vi "List Controls.vi"(8 "error in (no error)":errorcluster, 11 "Rename in":refnum<class "ProjectItem.lvclass">) -> (0 "error out":errorcluster, 3 "Rename out":refnum<class "ProjectItem.lvclass">)   [LabVIEW 2019, in "ProjectItem.lvclass"]
uses:
  ProjectItem.lvclass
  ProjectItem.lvclass/ProjectItem.ctl
  <vilib>/regexp/Match Regular Expression.xnode
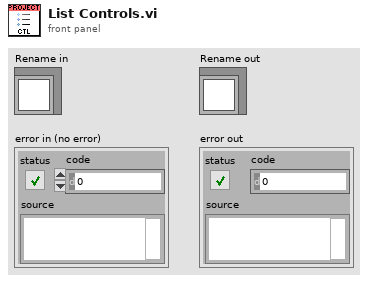
[diagram p1: front panel]
types:
  T1 = cluster{"Class":refnum<vi>, "DynamicVIs":refnum<vi>[], "StaticVIs":refnum<vi>[], "Controls":refnum<vi>[], "Name":string, "Icon":refnum<class "Icon.lvclass">}[]
  T2 = cluster{"Class":refnum<vi>, "DynamicVIs":refnum<vi>[], "StaticVIs":refnum<vi>[], "Controls":refnum<vi>[], "Name":string, "Icon":refnum<class "Icon.lvclass">}
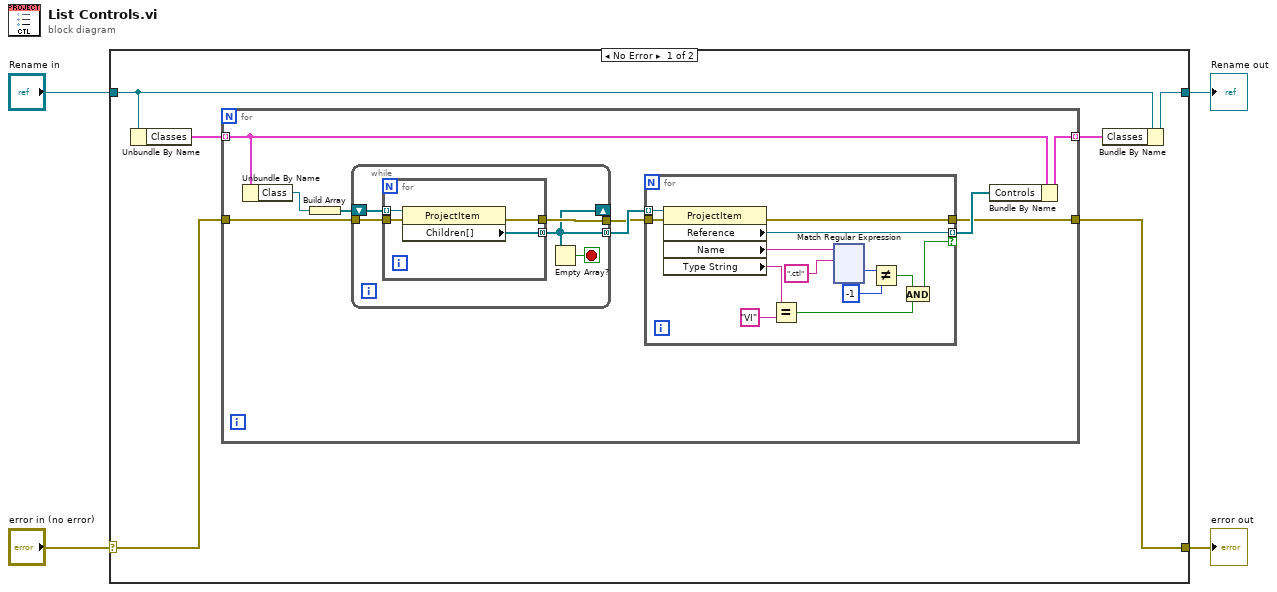
[diagram p0: block diagram]
diagram:
  n1 = case shown="No Error" "error in (no error)" {
    selector: "error in (no error)" -> [w6 w157]
    tunnel: [w9 w156] -> w4
    tunnel: "Rename in" -> [w8 w156]
    tunnel: [w5 w157] -> w2
    frame No Error {
      n2 = Unbundle By Name(w8) -> ("Classes"=w7:T1)
      n3 = for {
        tunnel: w7 -> [w19] mode=indexing
        tunnel: w6 -> [w13]
        tunnel: [w11] -> w5
        tunnel: [w18] -> w10 mode=indexing
        n4 = Unbundle By Name(w19) -> ("Class"=w17:refnum<vi>)
        n5 = Build Array(w17) -> (w16:refnum<vi>[])
        n6 = while {
          shift-right: [w147] -> _
          shift-left: w16 -> [w151]
          tunnel: [w147] -> w15 mode=concatenating
          tunnel: w13 -> [w149]
          tunnel: [w148] -> w12
          stop <- w150 stop-if-true
          n7 = for {
            tunnel: w151 -> [w155] mode=indexing
            tunnel: [w154] -> w147 mode=concatenating
            tunnel: w149 -> [w153]
            tunnel: [w152] -> w148
            n8 = property class="ProjectItem"(reference=w155, error in=w153) -> (error out=w152:errorcluster, "Children[]"=w154:refnum<vi>[])  [unwired: 1 out]
          }
          n9 = Empty Array?(array=w147) -> (empty?=w150:bool)
        }
        n10 = for {
          tunnel: w15 -> [w32] mode=indexing
          tunnel: [w27] -> w14 mode=indexing if=w24
          tunnel: w12 -> [w26]
          tunnel: [w25] -> w11
          n11 = property class="ProjectItem"(reference=w32, error in=w26) -> (error out=w25:errorcluster, "Reference"=w27:refnum<vi>, "Name"=w31:string, "Type String"=w23:string)  [unwired: 1 out]
          n12 = Equal?(x=w23, y="VI") -> (x = y?=w21:bool)
          n13 = xnode "Match Regular Expression"("input string"=w31, "regular expression"=".ctl") -> ("offset past match"=w29:i32)  [unwired: 4 in, 4 out]
          n14 = Not Equal?(x=w29, y=-1) -> (x != y?=w20:bool)
          n15 = And(x=w20, y=w21) -> (x .and. y?=w24:bool)
        }
        n16 = Bundle By Name(cluster=w19, "Controls"=w14) -> (w18:T2)
      }
      n17 = Bundle By Name(cluster=w8, "Classes"=w10) -> (w9:refnum<class "ProjectItem.lvclass">)
    }
    frame Error {
    }
  }
  "Rename out" <- w4
  "error out" <- w2
